vi "Set speed.vi"(10 "speed":dbl, 11 "shooter in":refnum<class "shooter.lvclass">) -> (3 "shooter out":refnum<class "shooter.lvclass">)   [LabVIEW 2015, in "shooter.lvclass"]
uses:
  shooter.lvclass
  shooter.lvclass/shooter.ctl
  Robot Global Data.vi
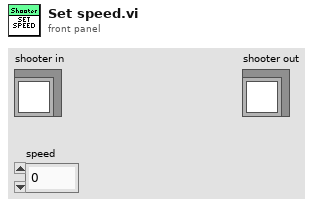
[diagram p1: front panel]
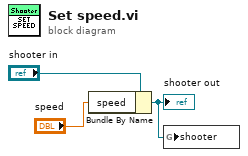
[diagram p0: block diagram]
diagram:
  n1 = Bundle By Name(cluster="shooter in", "speed"="speed") -> (w1:refnum<class "shooter.lvclass">)
  "shooter out" <- w1
  n2 = global write "Robot Global Data.vi" "shooter"(w1) -> ()
